vi "RH_DCPower_ConfigureSequenceCurrent.vi"(7 "DCPower_SequenceParameters":T1 {"DeltaVoltage" format="%.6p"; "DeltaTime" format="%.6p"; "Voltage Stop" format="%.6p"; "Aperture_time" format="%.6p"; "Current_range" format="%.6p"; "Current" format="%.6p"; "Voltage_range" format="%.6p"; "Voltage Start" format="%.6p"}, 8 "error in (no error)":errorcluster, 9 "Peak duration (s)":dbl, 10 "channel name":string, 11 "DCPower Session In":refnum<k15>) -> (0 "error out":errorcluster, 1 "num points":i32, 3 "DCPower Session Out":refnum<k15>)   [LabVIEW 2023, in "ResourceHandling.lvlib"]
doc: "Configure the SMU in Current Sequence Mode setting also the Aperture Time"
uses:
  ResourceHandling.lvlib
  TypeDefs/RH_DCPower_SequenceParameters.ctl
  <instrlib>/niDCPower/nidcpower.llb/niDCPower Output Function.ctl
  <instrlib>/niDCPower/nidcpower.llb/niDCPower Source Mode.ctl
  <instrlib>/niDCPower/nidcpower.llb/niDCPower Aperture Time Units.ctl
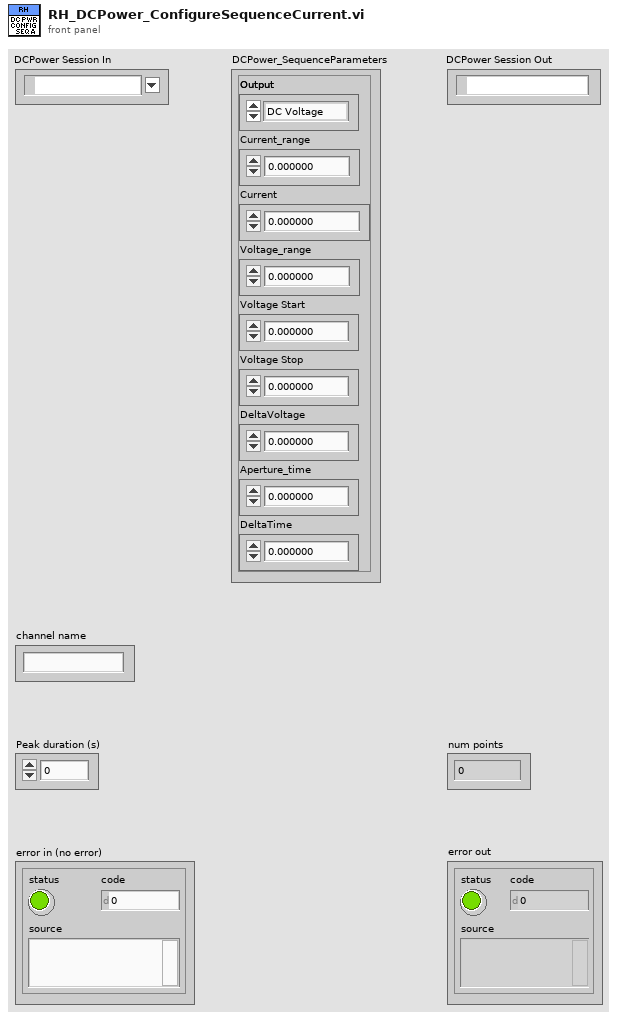
[diagram p1: front panel]
types:
  T1 = typedef "ResourceHandling.lvlib/RH_DCPower_SequenceParameters.ctl" = cluster{"Output":enum16{"DC Voltage", "DC Current"}, "Current_range":dbl, "Current":dbl, "Voltage_range":dbl, "Voltage Start":dbl, "Voltage Stop":dbl, "DeltaVoltage":dbl, "Aperture_time":dbl, "DeltaTime":dbl}
  T2 = typedef "niDCPower Source Mode.ctl" = i32
  T3 = typedef "niDCPower Output Function.ctl" = i32
  T4 = typedef "niDCPower Aperture Time Units.ctl" = i32
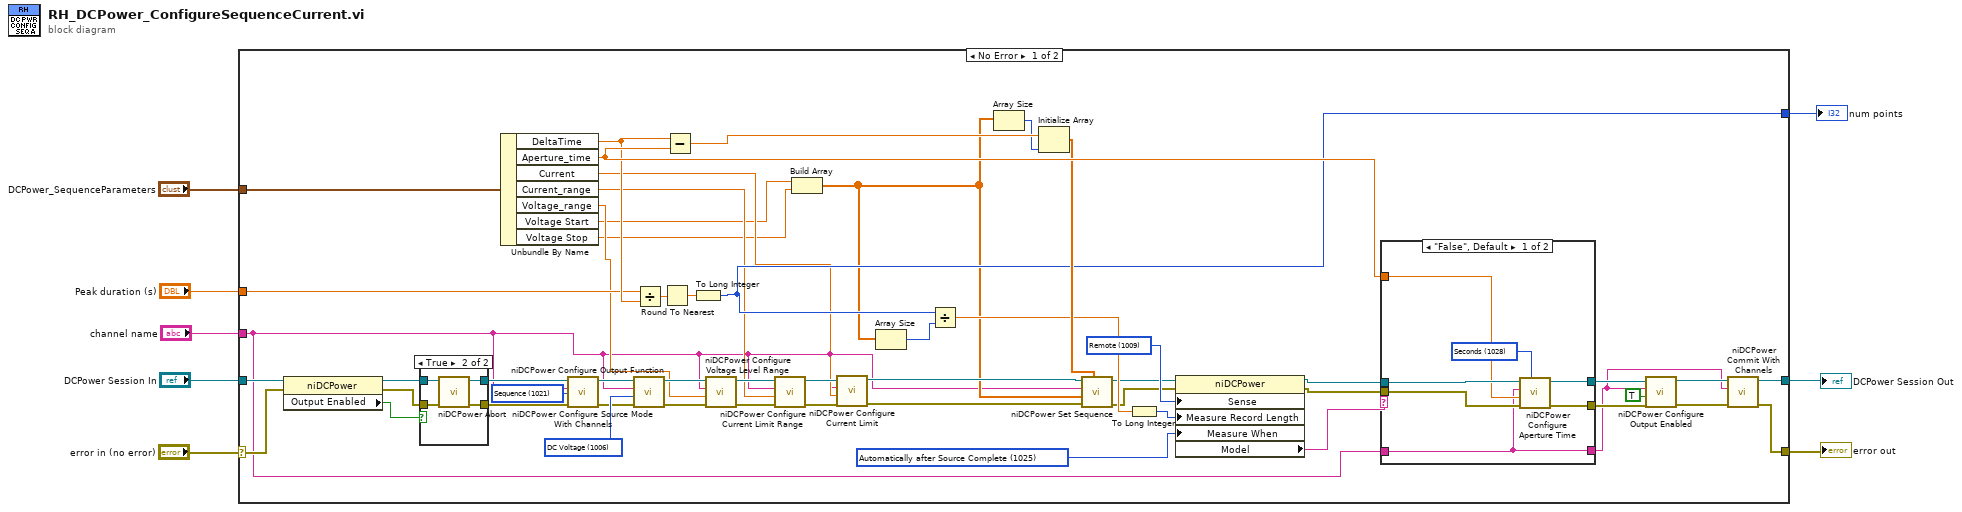
[diagram p0: block diagram]
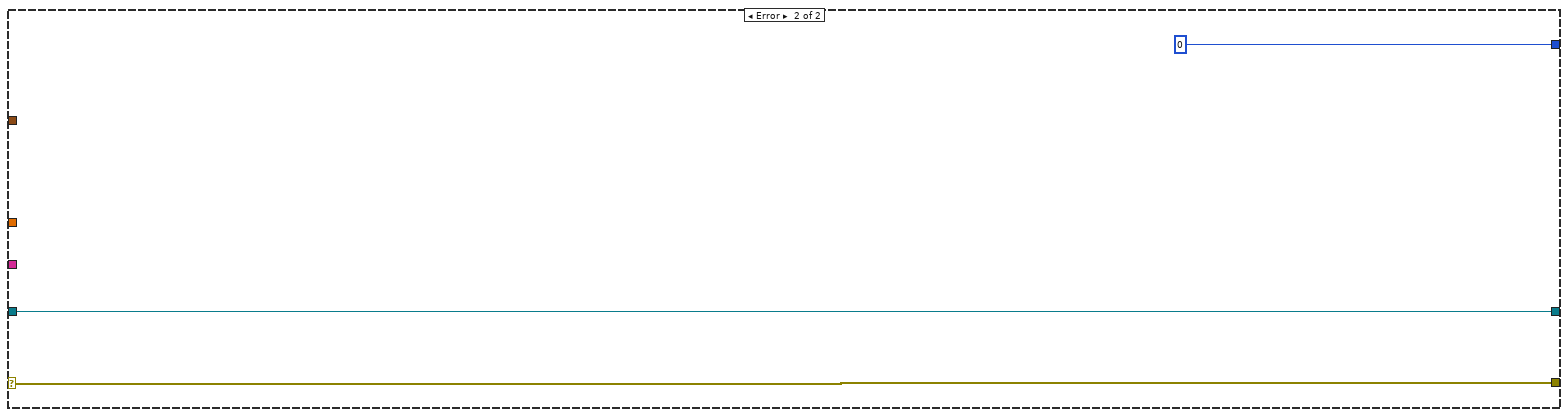
[diagram p4: hidden frame]
diagram:
  n1 = case shown="No Error" "error in (no error)" {
    selector: "error in (no error)" -> [w54 w80]
    tunnel: "DCPower Session In" -> [w55 w79]
    tunnel: "channel name" -> [w11 _]
    tunnel: "DCPower_SequenceParameters" -> [w49 _]
    tunnel: "Peak duration (s)" -> [w44 _]
    tunnel: [w39 0] -> w4
    tunnel: [w12 w80] -> w3
    tunnel: [w9 w79] -> w1
    frame No Error {
      w35 = 1009 items=["Local"=1008, "Remote"=1009] ("Measurement:Sense")
      w34 = 1025 items=["Automatically after Source Complete"=1025, "On Demand"=1026, "On Measure Trigger"=1027] ("Measurement:Advanced:Measure When")
      w50 = T2 1021 items=["Single Point"=1020, "Sequence"=1021] ("source mode")
      w53 = T3 1006 items=["DC Voltage"=1006, "DC Current"=1007, "Pulse Voltage"=1049, "Pulse Current"=1050] ("output function")
      n2 = property class="niDCPower"(reference=w55, error in=w54) -> (reference out=w61:refnum<k15>, error out=w62:errorcluster, "Output Enabled"=w60:bool)
      n3 = case shown="True" w60 {
        tunnel: w61 -> [w74 w78]
        tunnel: w62 -> [w73 w77]
        tunnel: [w74 w76] -> w51
        tunnel: [w73 w75] -> w52
        frame False {
        }
        frame True {
          n4 = call <instrlib>:"niDCPower Abort.vi"("error in (no error)"=w77, "instrument handle"=w78) -> ("error out"=w75:errorcluster, "instrument handle out"=w76:refnum<k15>)  [unwired: 8 in]
        }
      }
      n5 = Unbundle By Name(w49) -> ("DeltaTime"=w45:dbl, "Aperture_time"=w48:dbl, "Current"=w18:dbl, "Current_range"=w19:dbl, "Voltage_range"=w20:dbl, "Voltage Start"=w17:dbl, "Voltage Stop"=w16:dbl)
      n6 = call <instrlib>:"niDCPower Configure Source Mode With Channels.vi"("error in (no error)"=w52, "source mode"=w50, "channel name"=w11, "instrument handle"=w51) -> ("error out"=w38:errorcluster, "instrument handle out"=w37:refnum<k15>)  [unwired: 6 in]
      n7 = call <instrlib>:"niDCPower Configure Output Function.vi"("error in (no error)"=w38, "output function"=w53, "channel name"=w11, "instrument handle"=w37) -> ("error out"=w27:errorcluster, "instrument handle out"=w28:refnum<k15>)  [unwired: 6 in]
      n8 = Divide(x=w44, y=w45) -> (x/y=w43:dbl)
      n9 = Round To Nearest(number=w43) -> (nearest integer value=w42:dbl)
      n10 = Subtract(x=w45, y=w48) -> (x-y=w47:dbl)
      n11 = To Long Integer(number=w42) -> (32bit integer=w39:i32)
      n12 = call <instrlib>:"niDCPower Configure Voltage Level Range.vi"("error in (no error)"=w27, "voltage level range"=w20, "channel name"=w11, "instrument handle"=w28) -> ("error out"=w25:errorcluster, "instrument handle out"=w26:refnum<k15>)  [unwired: 6 in]
      n13 = call <instrlib>:"niDCPower Configure Current Limit Range.vi"("error in (no error)"=w25, "current limit range"=w19, "channel name"=w11, "instrument handle"=w26) -> ("error out"=w23:errorcluster, "instrument handle out"=w24:refnum<k15>)  [unwired: 6 in]
      n14 = Build Array(w17, w16) -> (w15:dbl[])
      n15 = call <instrlib>:"niDCPower Configure Current Limit.vi"("error in (no error)"=w23, "current limit"=w18, "channel name"=w11, "instrument handle"=w24) -> ("error out"=w22:errorcluster, "instrument handle out"=w21:refnum<k15>)  [unwired: 6 in]
      n16 = Array Size(array=w15) -> (size(s)=w14:i32)
      n17 = Divide(x=w39, y=w14) -> (x/y=w40:dbl)
      n18 = Array Size(array=w15) -> (size(s)=w41:i32)
      n19 = Initialize Array(w47, w41) -> (w46:dbl[])
      n20 = call <instrlib>:"niDCPower Set Sequence.vi"("source delays"=w46, "error in (no error)"=w22, "values"=w15, "channel name"=w11, "instrument handle"=w21) -> ("error out"=w32:errorcluster, "instrument handle out"=w33:refnum<k15>)  [unwired: 5 in]
      n21 = To Long Integer(number=w40) -> (32bit integer=w36:i32)
      n22 = property class="niDCPower"(reference=w33, error in=w32, "Sense"=w35, "Measure Record Length"=w36, "Measure When"=w34) -> (reference out=w30:refnum<k15>, error out=w29:errorcluster, "Model"=w31:string)
      n23 = case shown="\"False\", Default" w31 {
        tunnel: w30 -> [w69 w72]
        tunnel: w29 -> [w68 w71]
        tunnel: [w67 w71] -> w57
        tunnel: [w66 w72] -> w56
        tunnel: w48 -> [w65 _]
        tunnel: w11 -> [w63 w70]
        tunnel: [w63 w70] -> w10
        frame "False", Default {
          w64 = T4 1028 items=["Seconds"=1028, "Powerline Cycles"=1029] ("aperture time units")
          n24 = call <instrlib>:"niDCPower Configure Aperture Time.vi"("aperture time units"=w64, "error in (no error)"=w68, "aperture time"=w65, "channel name"=w63, "instrument handle"=w69) -> ("error out"=w67:errorcluster, "instrument handle out"=w66:refnum<k15>)  [unwired: 5 in]
        }
        frame "NI PXI-4110" {
        }
      }
      n25 = call <instrlib>:"niDCPower Configure Output Enabled.vi"("error in (no error)"=w57, "output enabled"=TRUE, "channel name"=w10, "instrument handle"=w56) -> ("error out"=w59:errorcluster, "instrument handle out"=w58:refnum<k15>)  [unwired: 6 in]
      n26 = call <instrlib>:"niDCPower Commit With Channels.vi"("error in (no error)"=w59, "channel name"=w10, "instrument handle"=w58) -> ("error out"=w12:errorcluster, "instrument handle out"=w9:refnum<k15>)  [unwired: 7 in]
    }
    frame Error {
    }
  }
  "error out" <- w3
  "num points" <- w4
  "DCPower Session Out" <- w1
